vi "Probe Information.vi"(11 "Gesture in":refnum<class "Gesture.lvclass">) -> (2 "probe information":string)   [LabVIEW 2023, in "Gesture.lvclass"]
doc: "Generate the string that is used to display gesture information in the probe window."
uses:
  Gesture.lvclass
  Gesture.lvclass/Gesture.ctl
panel:
  in  "format string":string="%d milliseconds\nMouse gesture: %s\nPoint: (%f, %f)\nOffset: (%f, %f)"
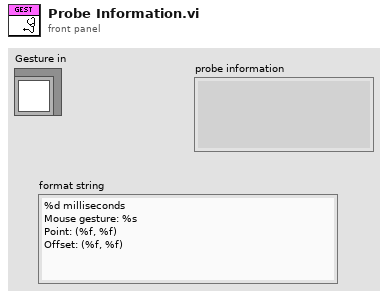
[diagram p1: front panel]
types:
  T1 = typedef "Gesture.lvclass/Gesture Enum.ctl" = enum16{"None", "Stop", "Tap", "Press", "Pan Start", "Pan Continue", "Pan End", "Pinch Open", "Pinch Close", "Double Tap"}
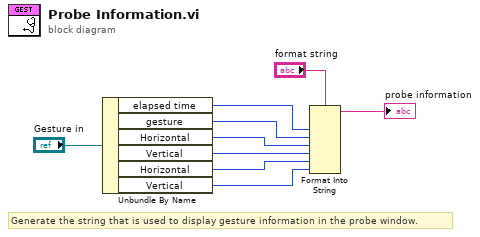
[diagram p0: block diagram]
diagram:
  # "Generate the string that is used to display gesture information in the probe window."
  n1 = Unbundle By Name("Gesture in") -> ("elapsed time"=w8:u32, "gesture"=w7:T1, "Horizontal"=w6:i32, "Vertical"=w5:i32, "Horizontal"=w4:i32, "Vertical"=w3:i32)
  n2 = Format Into String(format string="format string", w8, w7, w6, w5, w4, w3) -> (resulting string=→"probe information":string)  [unwired: 2 in, 1 out]
